vi "toString.vi"(7 "UTC? (F)":bool, 9 "Timestamp (now)":timestamp, 11 "DateTime.RFC5322 in":refnum<class "DateTime.RFC5322.lvclass">) -> (1 "DateTime String":string, 3 "DateTime.RFC5322 out":refnum<class "DateTime.RFC5322.lvclass">)   [LabVIEW 2013, in "DateTime.RFC5322.lvclass"]
uses:
  DateTime.RFC5322.lvclass
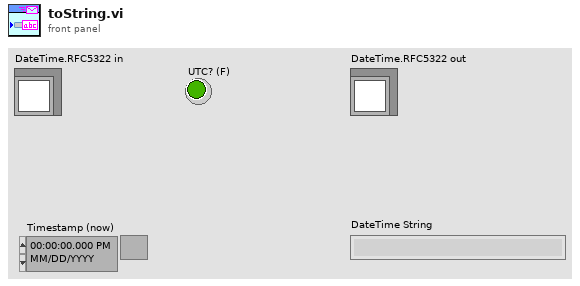
[diagram p1: front panel]
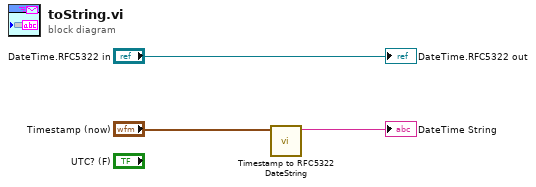
[diagram p0: block diagram]
diagram:
  n1 = call "Timestamp to RFC5322 DateString.vi"("Timestamp (now)"="Timestamp (now)") -> ("RFC5322 Date String"=→"DateTime String":string)  [unwired: 10 in]
  "DateTime.RFC5322 out" <- "DateTime.RFC5322 in"
